vi "LUnit Configure.vi"(8 "error in (no error)":errorcluster, 9 "Default Path":path, 10 "Interactive?":bool, 11 "Coverage Report In":refnum<class "Coverage Report.lvclass">) -> (0 "error out":errorcluster, 3 "Coverage Report Out":refnum<class "Coverage Report.lvclass">)   [LabVIEW 2020, in "Coverage Report.lvclass"]
uses:
  Coverage Report.lvclass
  Coverage Report.lvclass/Coverage Report.ctl
  <vilib>/Astemes/LUnit/Framework/Configuration Manager/LUnit Configuration Manager.lvclass
  f97740a0-8655-44de-873d-fc598e584b33.vi
panel:
  in  "VI tree":string[](tree)
  out "Coverage Include File Path":path
  in  "Cancel":bool
  in  "Commit":bool
  in  "Open New Reports":bool
  in  "Report Path":path
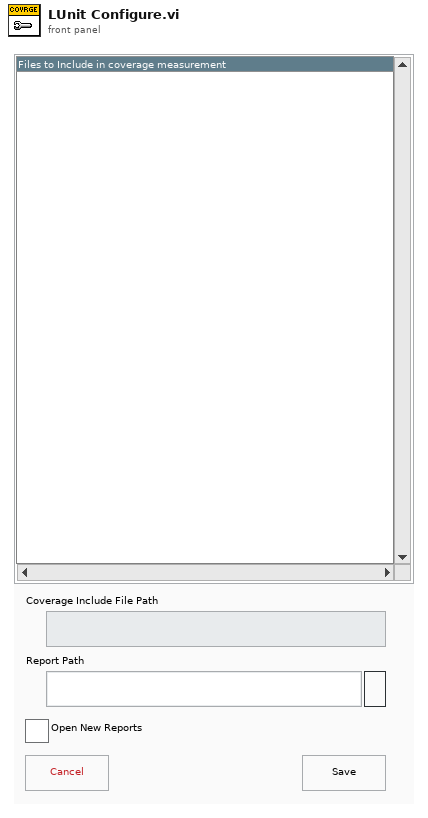
[diagram p1: front panel]
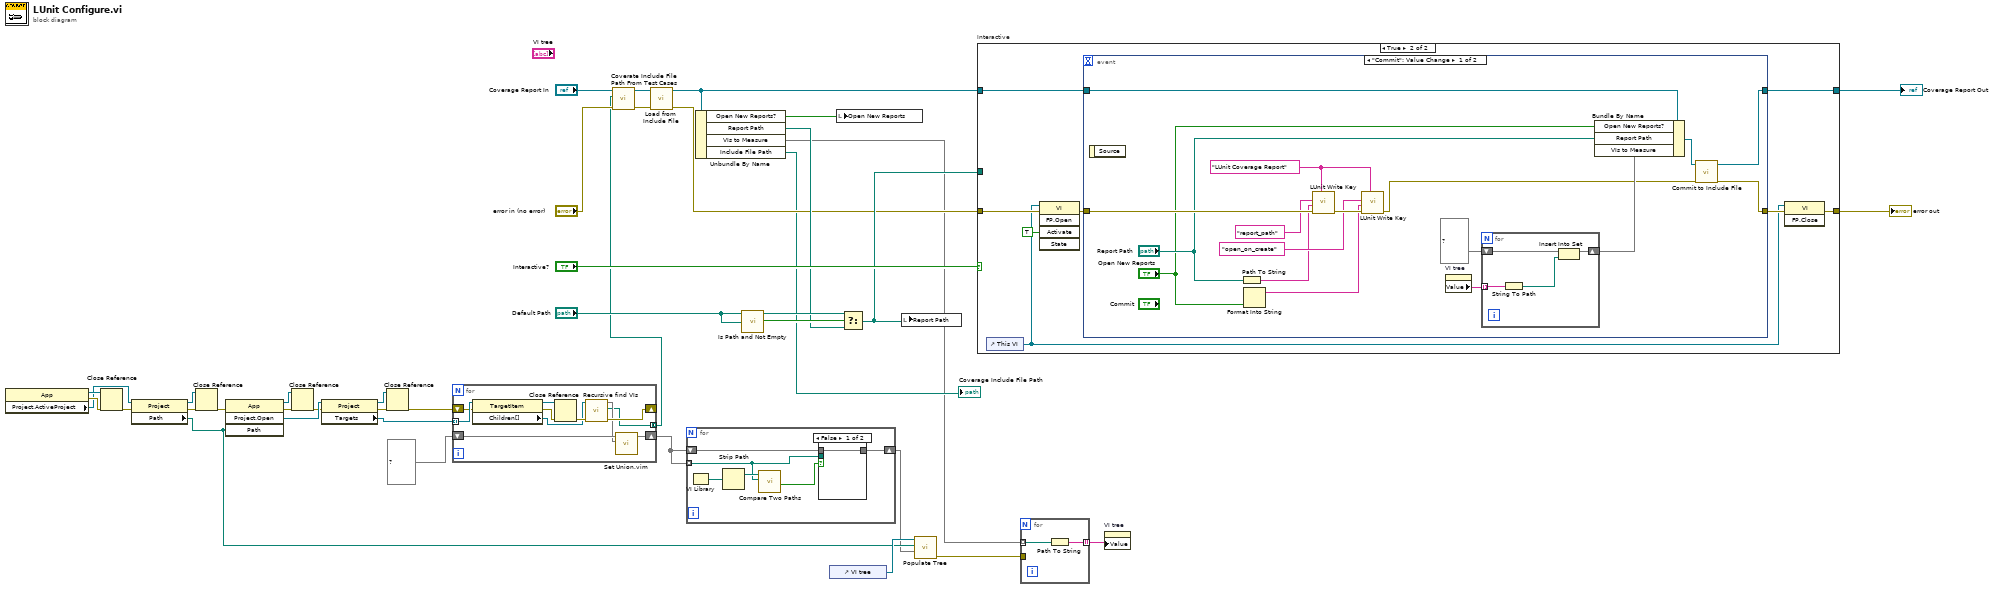
[diagram p0: block diagram]
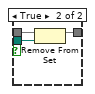
[diagram p2: hidden frame]
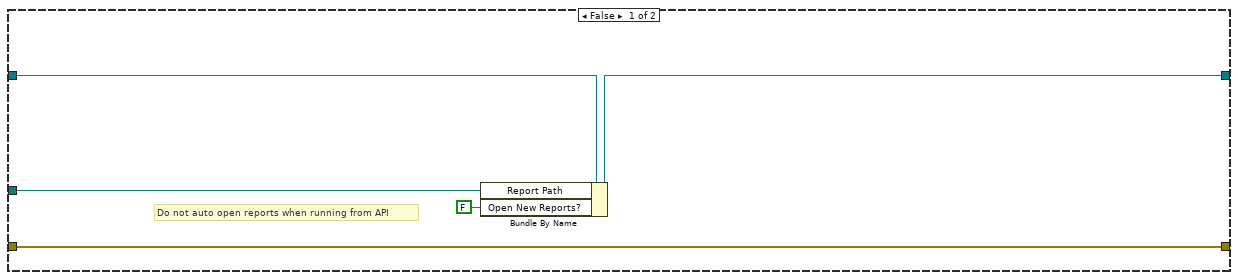
[diagram p3: hidden frame]
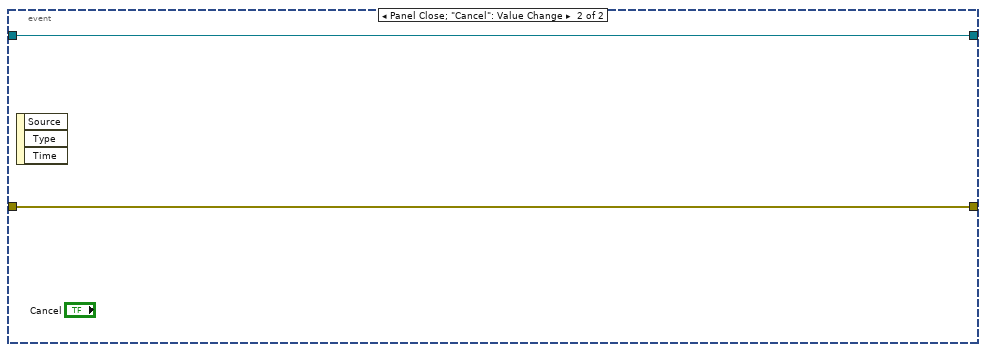
[diagram p4: hidden frame]
diagram:
  n1 = property class="App"() -> (reference out=w17:refnum<vi>, error out=w20:errorcluster, "Project.ActiveProject"=w16:refnum<vi>)  [unwired: 2 in]
  n2 = Close Reference(reference=w17, error in (no error)=w20) -> (error out=w21:errorcluster)
  n3 = property class="Project"(reference=w16, error in=w21) -> (reference out=w18:refnum<vi>, error out=w19:errorcluster, "Path"=w3:path)
  n4 = Close Reference(reference=w18, error in (no error)=w19) -> (error out=w22:errorcluster)
  n5 = invoke class="App" method="Project.Open"(error in=w22, "Path"=w3) -> (reference out=w25:refnum<vi>, error out=w29:errorcluster, "Project:Open"=w31:refnum<vi>)  [unwired: 2 in, 1 out]
  n6 = Close Reference(reference=w25, error in (no error)=w29) -> (error out=w26:errorcluster)
  n7 = property class="Project"(reference=w31, error in=w26) -> (reference out=w27:refnum<vi>, error out=w30:errorcluster, "Targets"=w23:refnum<vi>[])
  n8 = Close Reference(reference=w27, error in (no error)=w30) -> (error out=w28:errorcluster)
  n9 = for {
    tunnel: w23 -> [w50] mode=indexing
    shift-right: [w47] -> _
    shift-left: w28 -> [w48]
    shift-right: [w43] -> w6
    shift-left: set{path} {} ("VIs") -> [w45]
    tunnel: [w40] -> w9 mode=concatenating
    n10 = property class="TargetItem"(reference=w50, error in=w48) -> (reference out=w46:refnum<vi>, error out=w49:errorcluster, "Children[]"=w41:refnum<vi>[])
    n11 = Close Reference(reference=w46, error in (no error)=w49) -> (error out=w42:errorcluster)
    n12 = call "Recursive find VIs.vi"("error in (no error)"=w42, "Project Items"=w41) -> ("error out"=w47:errorcluster, "Test Case Classes"=w40:path[], "VIs"=w44:set{path})  [unwired: 7 in]
    n13 = call "Set Union.vim"("set 2"=w44, "set 1"=w45) -> ("union"=w43:set{path})  [unwired: 9 in]
  }
  n14 = call "Coverate Include File Path From Test Cases.vi"("error in (no error)"="error in (no error)", "Test Case Classes"=w9, "Coverage Report.lvclass"="Coverage Report In") -> ("error out"=w14:errorcluster, "Coverage Report.lvclass 2"=w15:refnum<class "Coverage Report.lvclass">)  [unwired: 7 in]
  n15 = call "Load from Include File.vi"("error in (no error)"=w14, "Coverage Report in"=w15) -> ("error out"=w10:errorcluster, "Coverage Report out"=w12:refnum<class "Coverage Report.lvclass">)  [unwired: 8 in]
  n16 = for {
    tunnel: w6 -> [w53] mode=indexing
    shift-right: [w52] -> w2
    shift-left: w6 -> [w54]
    n17 = VI Library() -> (path=w55:path)
    n18 = Strip Path(path=w55) -> (stripped path=w56:path)  [unwired: 1 out]
    n19 = call <vilib>:"Compare Two Paths.vi"("Path 2"=w53, "Path 1"=w56) -> ("Path 2 Relative to Path 1?"=w51:bool)  [unwired: 6 in, 3 out]
    n20 = case shown="False" w51 {
      tunnel: w54 -> [w57 w60]
      tunnel: w53 -> [_ w59]
      tunnel: [w57 w58] -> w52
      frame False {
      }
      frame True {
        n21 = Remove From Set(10:w59, 11:w60) -> (3:w58:set{path})  [unwired: 1 out]
      }
    }
  }
  n22 = Unbundle By Name(w12) -> ("Open New Reports?"=w32:bool, "Report Path"=w33:path, "VIs to Measure"=w4:set{path}, "Include File Path"=→"Coverage Include File Path":path)
  n23 = call <vilib>:"Is Path and Not Empty.vi"("path"="Default Path") -> ("Is Path and Not Empty?"=w36:bool)  [unwired: 4 in]
  n24 = control-ref of="VI tree"() -> (w7:refnum<vi>)
  n25 = local write "Open New Reports"(w32) -> ()
  n26 = Select(t="Default Path", s=w36, f=w33) -> (s? t:f=w35:path)
  n27 = local write "Report Path"(w35) -> ()
  n28 = call "Populate Tree.vi"("VIs"=w2, "Project Path"=w3, "TreeControl in"=w7) -> ("error out"=w1:errorcluster)  [unwired: 8 in]
  n29 = case "Interactive" shown="True" "Interactive?" {
    tunnel: w10 -> [w65 w71]
    tunnel: [w65 w69] -> w39
    tunnel: w12 -> [w64 w66]
    tunnel: [w63 w67] -> w37
    tunnel: w35 -> [w62 _]
    frame False {
      # "Do not auto open reports when running from API"
      n30 = Bundle By Name(cluster=w64, "Report Path"=w62, "Open New Reports?"=FALSE) -> (w63:refnum<class "Coverage Report.lvclass">)
    }
    frame True {
      n31 = control-ref of="This VI"() -> (w68:refnum<vi>)
      n32 = invoke class="VI" method="FP.Open"(reference=w68, error in=w71, "Activate"=TRUE ("Activate?")) -> (error out=w72:errorcluster)  [unwired: 2 in, 4 out]
      n33 = event shown="[0] \"Commit\": Value Change" {
        selector: _ -> [_ _]
        dyn-events: _ -> [_ _]
        timeout: _ -> [_ _]
        tunnel: w72 -> [w90 w96]
        tunnel: [w77 w96] -> w70
        tunnel: w66 -> [w84 w95]
        tunnel: [w78 w95] -> w67
        event "Commit": Value Change {
          w75 = "LUnit Coverage Report"
          n34 = event-data() -> ()  [unwired: 1 in, 1 out]
          n35 = Path To String(path="Report Path") -> (string=w86:string)
          n36 = Format Into String("Open New Reports") -> (resulting string=w85:string)  [unwired: 3 in, 1 out]
          n37 = call <vilib>:"LUnit Write Key.vi"("section"=w75, "error in (no error)"=w90, "value"=w86, "key"="report_path" ("Name")) -> ("error out"=w89:errorcluster)  [unwired: 7 in]
          n38 = call <vilib>:"LUnit Write Key.vi"("section"=w75, "error in (no error)"=w89, "value"=w85, "key"="open_on_create" ("Name")) -> ("error out"=w76:errorcluster)  [unwired: 7 in]
          n39 = property on="VI tree" class="Tree (strict)"() -> ("Value"=w74:string[])  [unwired: 2 in, 2 out]
          n40 = for {
            shift-right: [w93] -> w79
            shift-left: set{path} {} ("VIs to Measure") -> [w94]
            tunnel: w74 -> [w92] mode=indexing
            n41 = String To Path(string=w92) -> (path=w91:path)
            n42 = Insert Into Set(10:w91, 11:w94) -> (3:w93:set{path})  [unwired: 1 out]
          }
          n43 = Bundle By Name(cluster=w84, "Open New Reports?"="Open New Reports", "Report Path"="Report Path", "VIs to Measure"=w79) -> (w83:refnum<class "Coverage Report.lvclass">)
          n44 = call "Commit to Include File.vi"("error in (no error)"=w76, "Coverage Report in"=w83) -> ("error out"=w77:errorcluster, "Coverage Report out"=w78:refnum<class "Coverage Report.lvclass">)  [unwired: 8 in]
        }
        event Panel Close; "Cancel": Value Change {
          n45 = event-data() -> ()  [unwired: 1 in, 3 out]
        }
      }
      n46 = invoke class="VI" method="FP.Close"(reference=w68, error in=w70) -> (error out=w69:errorcluster)  [unwired: 1 in, 2 out]
    }
  }
  "error out" <- w39
  "Coverage Report Out" <- w37
  n47 = for {
    tunnel: w4 -> [w98] mode=indexing
    tunnel: [w97] -> w5 mode=indexing
    tunnel: w1 -> [_]
    n48 = Path To String(path=w98) -> (string=w97:string)
  }
  n49 = property on="VI tree" class="Tree (strict)"("Value"=w5) -> ()  [unwired: 2 in, 2 out]
